vi "Set HIL Mode.vi"(7 "Box ID":i32, 8 "error in (no error)":errorcluster, 10 "Enable":bool, 11 "CAN in":refnum<class "XNET_BS120x.lvclass">) -> (0 "error out":errorcluster, 3 "CAN out":refnum<class "XNET_BS120x.lvclass">)   [LabVIEW 2021, in "BS120x Driver.lvlib" / "XNET_BS120x.lvclass"]
doc: "When in HIL mode, the Battery Simulator 1200 gives priority to the specified incoming frames to reduce latency; the instrument will attempt to pass non-HIL frames through for processing but delivery is not guaranteed.\n(c) 2019 Bloomy Controls, Inc. All rights reserved."
uses:
  XNET_BS120x.lvclass
  BS120x.lvclass
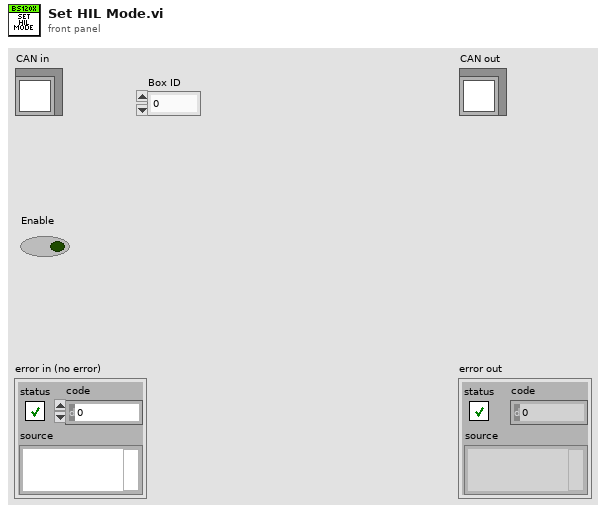
[diagram p1: front panel]
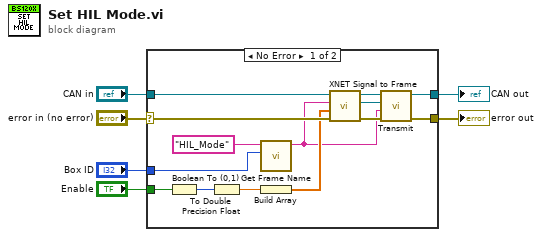
[diagram p0: block diagram]
diagram:
  n1 = case shown="No Error" "error in (no error)" {
    selector: "error in (no error)" -> [w16 w22]
    tunnel: [w17 w22] -> w5
    tunnel: [w10 w21] -> w3
    tunnel: "CAN in" -> [w11 w21]
    tunnel: "Enable" -> [w13 _]
    tunnel: "Box ID" -> [w8 _]
    frame No Error {
      n2 = Boolean To (0,1)(Boolean=w13) -> (0, 1=w14:i16)
      n3 = To Double Precision Float(number=w14) -> (double precision float=w15:dbl)
      n4 = call "Get Frame Name.vi"("Box ID"=w8, "Frame Name"="HIL_Mode" ("name")) -> ("Frame Name out"=w7:string)  [unwired: 9 in]
      n5 = Build Array(w15) -> (w12:dbl[])
      n6 = call "XNET Signal to Frame.vi"("error in (no error)"=w16, "Data Array"=w12, "Frame"=w7, "CAN in"=w11) -> ("error out"=w20:errorcluster, "Data"=w19:refnum<class "XNET Data.lvclass">, "CAN out"=w18:refnum<class "XNET_BS120x.lvclass">)  [unwired: 5 in]
      n7 = call "Transmit.vi"("error in (no error)"=w20, "Frame"=w7, "Data in"=w19, "CAN in"=w18) -> ("error out"=w17:errorcluster, "CAN out"=w10:refnum<class "XNET_BS120x.lvclass">)  [unwired: 6 in]
    }
    frame Error {
    }
  }
  "error out" <- w5
  "CAN out" <- w3
